vi "APC_9049_HRL_ZeroPhaseFIlter.vi"(2 "Init value compensation":bool, 3 "IIR Filter Cluster":T1, 4 "Pcyl":dbl[](array[numeric])) -> (0 "Pcylfilt":dbl[](array[numeric]), 1 "Pressure filtering":dbl[][](graph))   [LabVIEW 2020]
uses:
  <vilib>/Analysis/3filter.llb/Zero Phase Filter (Cascade, DBL).vi
  <vilib>/Analysis/NI_AALBase.lvlib
panel:
  in  "Graph":bool
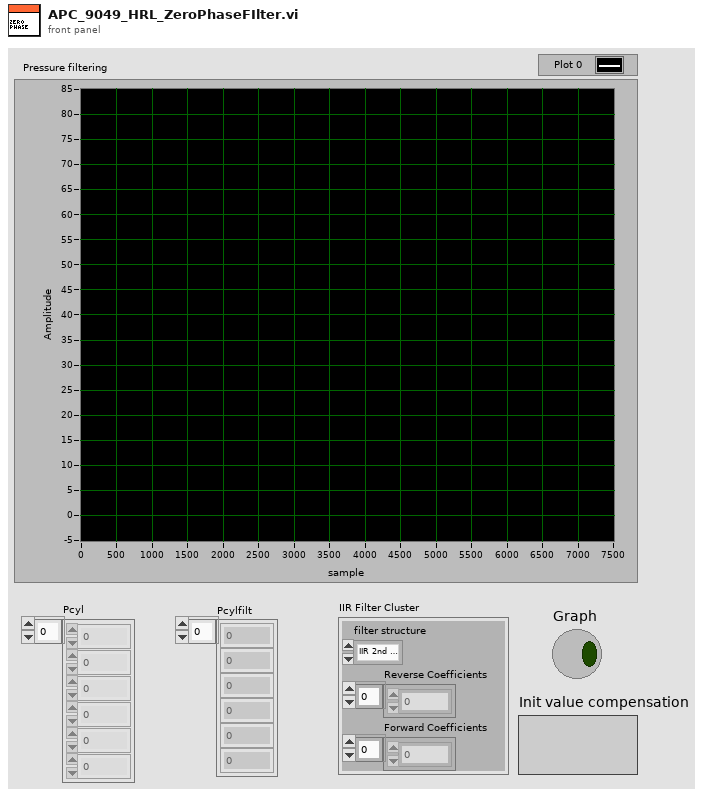
[diagram p1: front panel]
types:
  T1 = cluster{"filter structure":enum32{"IIR 2nd Order", "IIR 4th Order"}, "Reverse Coefficients":dbl[], "Forward Coefficients":dbl[]}
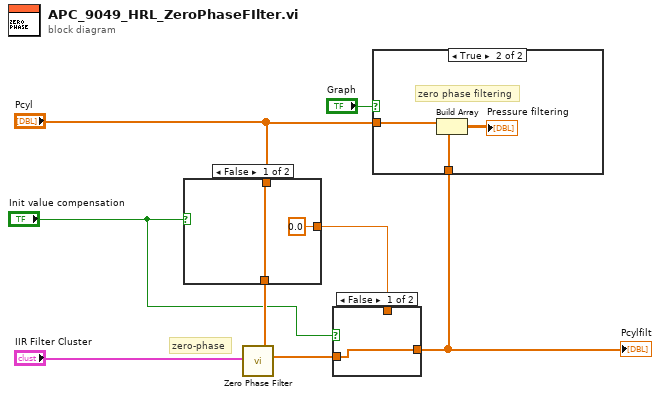
[diagram p0: block diagram]
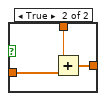
[diagram p2: hidden frame]
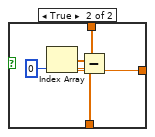
[diagram p3: hidden frame]
diagram:
  # "zero-phase"
  n1 = case shown="False" "Init value compensation" {
    tunnel: "Pcyl" -> [w10 w14]
    tunnel: [w10 w13] -> w5
    tunnel: [0.0 ("Numeric") w12] -> w3
    frame False {
    }
    frame True {
      n2 = Index Array(array=w14, index=0) -> (element=w12:dbl)
      n3 = Subtract(x=w14, y=w12) -> (x-y=w13:dbl[])
    }
  }
  n4 = call-poly <vilib>:"Zero Phase Filter.vi"("IIR Filter Cluster"="IIR Filter Cluster", "X"=w5) -> ("Filtered X"=w6:dbl[])  [unwired: 8 in, 1 out]
  n5 = case shown="False" "Init value compensation" {
    tunnel: [w15 w18] -> w7
    tunnel: w6 -> [w15 w17]
    tunnel: w3 -> [_ w16]
    frame False {
    }
    frame True {
      n6 = Add(x=w16, y=w17) -> (x+y=w18:dbl[])
    }
  }
  "Pcylfilt" <- w7
  n7 = case shown="True" "Graph" {
    tunnel: "Pcyl" -> [_ w21]
    tunnel: w7 -> [_ w20]
    frame False {
    }
    frame True {
      # "zero phase filtering"
      n8 = Build Array(w21, w20) -> (→"Pressure filtering":dbl[][])
    }
  }
